vi "웹서버 데이터 읽기.vi"(8 "에러 입력(에러 없음)":errorcluster, 11 "참조 번호 입력":T1 caption="client handle out") -> (0 "에러 출력":errorcluster, 2 "출력값":string, 3 "참조 번호 출력":T1 caption="client handle out")   [LabVIEW 2019]
uses:
  <vilib>/httpClient/ClientHandle.ctl
  <vilib>/httpClient/LabVIEWHTTPClient.lvlib
panel:
  out "headers":string caption="헤더"
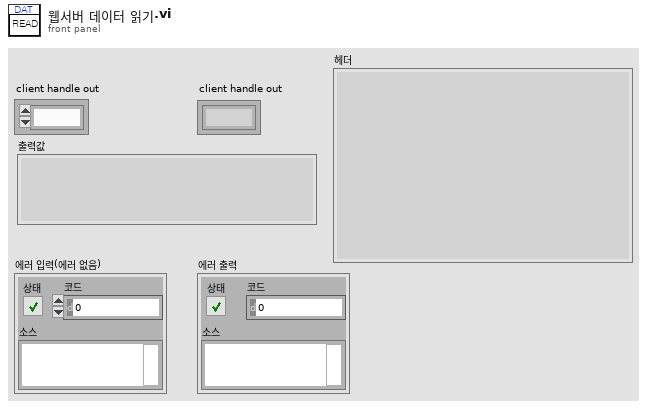
[diagram p1: front panel]
types:
  T1 = typedef "LabVIEWHTTPClient.lvlib/ClientHandle.ctl" = refnum<k1>
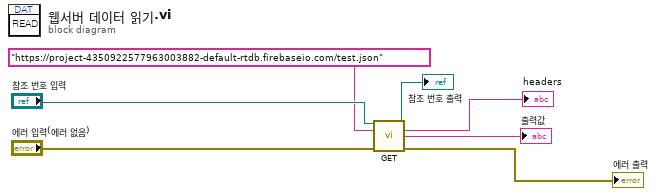
[diagram p0: block diagram]
diagram:
  n1 = call <vilib>:"GET.vi"("client handle"="참조 번호 입력", "url"="https://project-4350922577963003882-default-rtdb.firebaseio.com/test.json", "error in (no error)"="에러 입력(에러 없음)") -> ("client handle out"=→"참조 번호 출력":T1, "headers"=→"headers":string, "body"=→"출력값":string, "error out"=→"에러 출력":errorcluster)  [unwired: 9 in]
